vi "GetEnqueuer.vi"(8 "error in (no error)":errorcluster, 10 "Actor Name":string, 11 "TopLevel in":refnum<class "TopLevel.lvclass">) -> (0 "error out":errorcluster, 2 "Enqueuer":refnum<class "Message Enqueuer.lvclass">, 3 "TopLevel out":refnum<class "TopLevel.lvclass">)   [LabVIEW 2019, in "TopLevel.lvlib" / "TopLevel.lvclass"]
uses:
  TopLevel.lvclass
  <vilib>/ActorFramework/Message Enqueuer/Message Enqueuer.lvclass
  TopLevel.lvclass/TopLevel.ctl
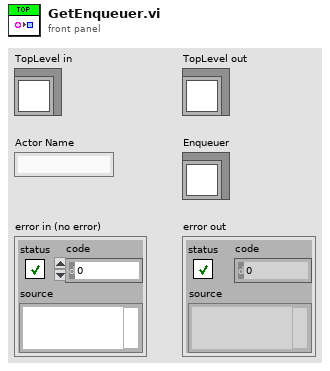
[diagram p1: front panel]
types:
  T1 = map{string, refnum<class "Message Enqueuer.lvclass">}
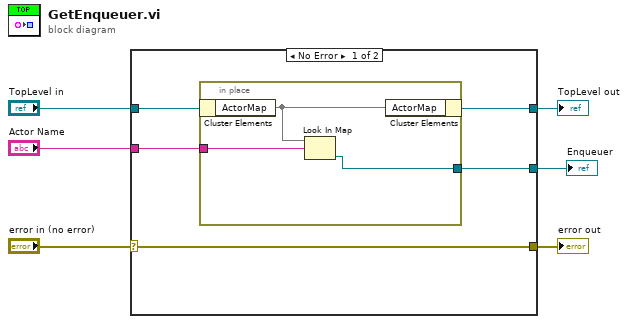
[diagram p0: block diagram]
diagram:
  n1 = case shown="No Error" "error in (no error)" {
    selector: "error in (no error)" -> [w7 w16]
    tunnel: [w7 w16] -> w5
    tunnel: [w10 w15] -> w3
    tunnel: "TopLevel in" -> [w11 w15]
    tunnel: "Actor Name" -> [w9 _]
    tunnel: [w8 _] -> w1
    frame No Error {
      n2 = in-place {
        in-place-border: w9 -> [w13]
        in-place-border: [w12] -> w8
        n3 = in-place-cluster #1(w11) -> ("ActorMap"=w14:T1)
        n4 = Look In Map(map=w14, key=w13) -> (value=w12:refnum<class "Message Enqueuer.lvclass">)  [unwired: 1 in, 1 out]
        n5 = in-place-cluster #1("ActorMap"=w14) -> (w10:refnum<class "TopLevel.lvclass">)
      }
    }
    frame Error {
    }
  }
  "error out" <- w5
  "TopLevel out" <- w3
  "Enqueuer" <- w1
